vi "Result Datam.vi"() -> ()   [LabVIEW 2012]
uses:
  <vilib>/Analysis/NI_AALPro.lvlib
panel:
  out "Graph Polarizer":cluster{dbl[], dbl[]}[](graph)
  in  "Polarizer and Analyser Scan":refnum<user-event>
  in  "Polarizer Scan":refnum<user-event>
  in  "Make this a motor null":refnum<user-event>
  in  "Panel Clouse and Stop":refnum<user-event>
  in  "Minimum Absolute Null":i32(listbox)
  in  "Table Absolute Null":i32(listbox)
  in  "Table Polarizer":i32(listbox)
  in  "Event Polarizer":refnum<user-event>
  in  "stop":bool
  out "XY Absolute Null":cluster{dbl[], dbl[]}[](graph)
  # "Polarizer"
  # "Absolute null"
  # "Minimum"
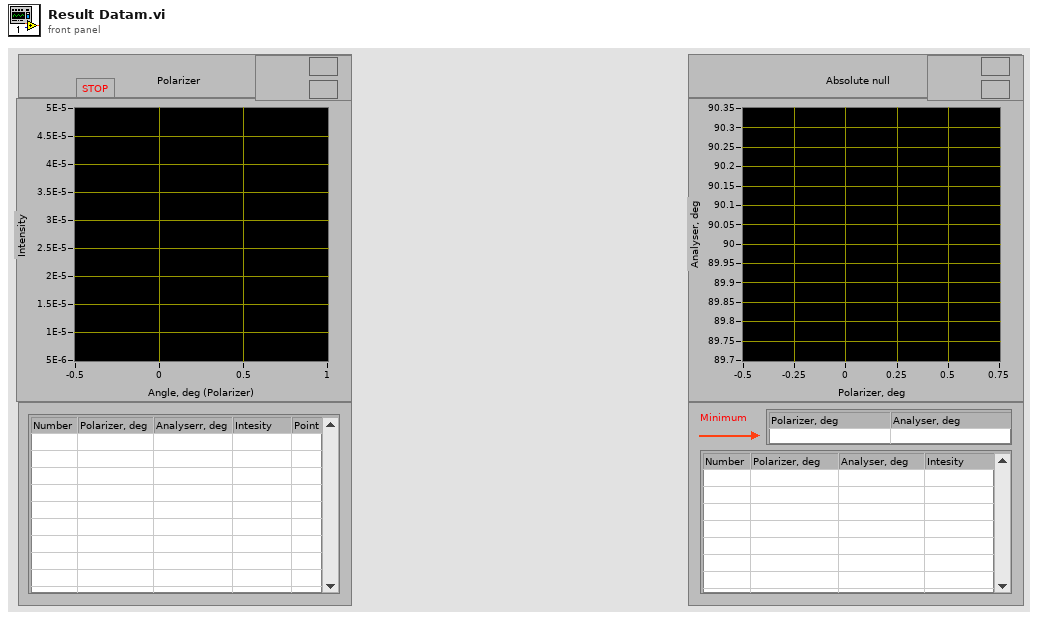
[diagram p1: front panel]
types:
  T1 = cluster{"Counter Pol":i32, "Counter A":i32, "Number Graph Pol":i32, "Number Graph A":i32, "Counter Abs Null":i32, "Pol Abs null deg":dbl, "A Abs null deg":dbl}
  T2 = cluster{"Kol-vo":i32, "Analyser":dbl, dbl[], dbl[], dbl[]}
  T3 = cluster{"Kol-vo":i32, "Analyser":dbl, dbl[], dbl[], dbl[]}[]
  T4 = cluster{"Kol-vo":i32, "Polarizer":dbl, dbl[], dbl[], dbl[]}
  T5 = cluster{"Kol-vo":i32, "Polarizer":dbl, dbl[], dbl[], dbl[]}[]
  T6 = enum32{"SVD", "Givens", "Givens2", "Householder", "LU Decomposition", "Cholesky"}
  T7 = cluster{"Pol Abs null deg":dbl, "A Abs null deg":dbl}
  T8 = cluster{"Kol-vo":i32, "Analyser":dbl, dbl[], dbl[], "Best Polynomial Fit":dbl[]}
  T9 = cluster{"Kol-vo":i32, "Polarizer":dbl, dbl[], dbl[], "Best Polynomial Fit":dbl[]}
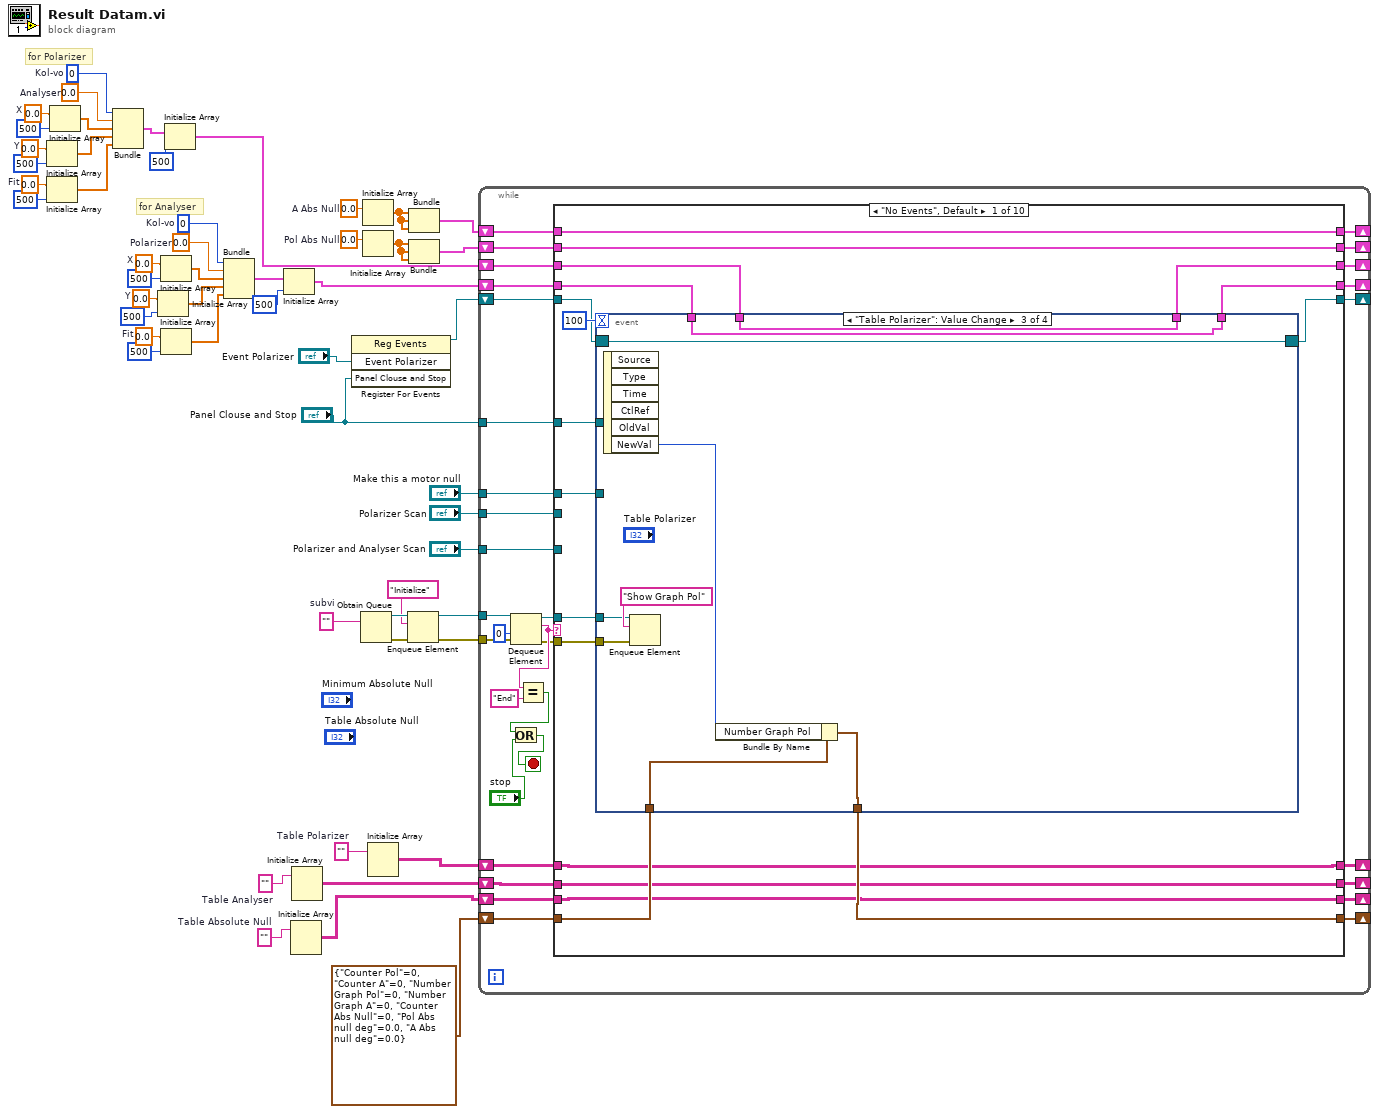
[diagram p0: block diagram]
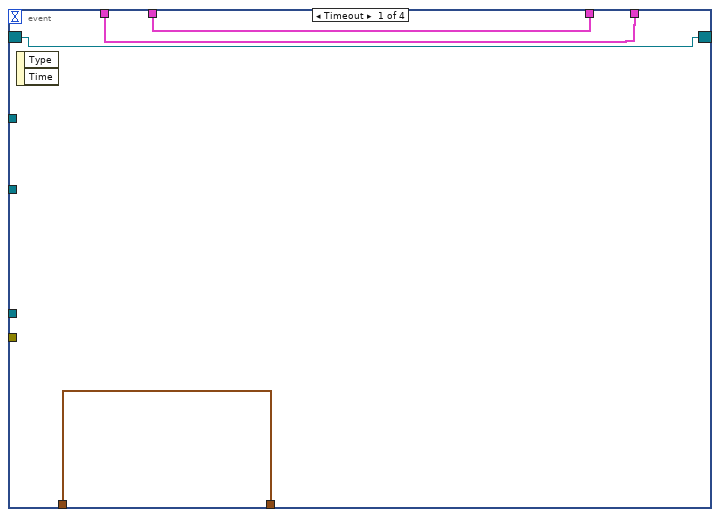
[diagram p2: hidden frame]
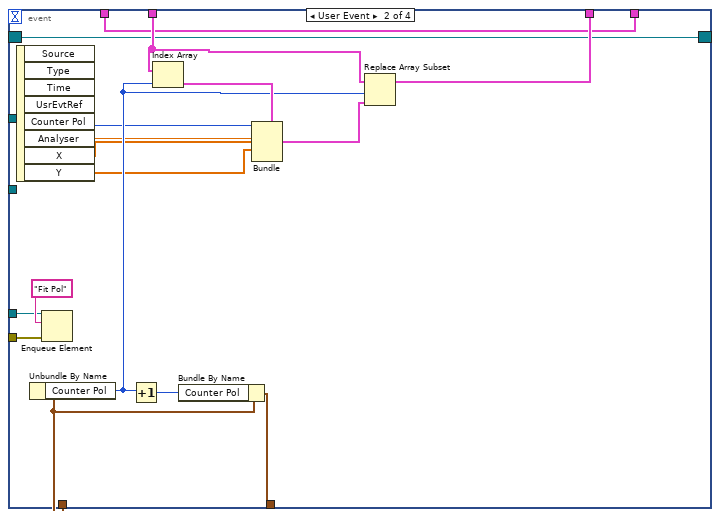
[diagram p3: hidden frame]
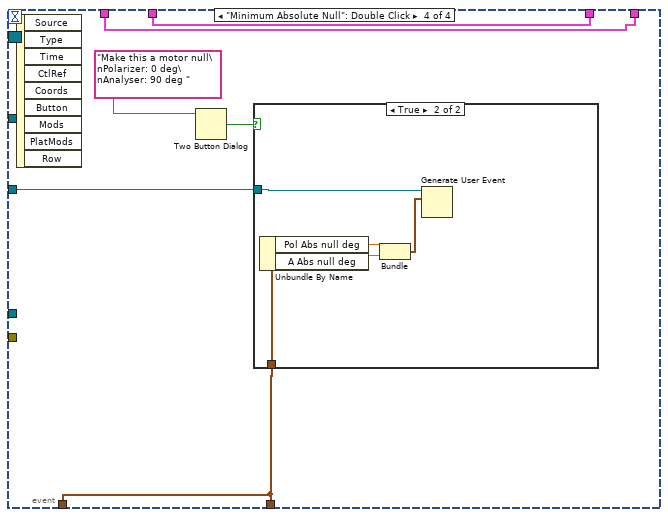
[diagram p4: hidden frame]
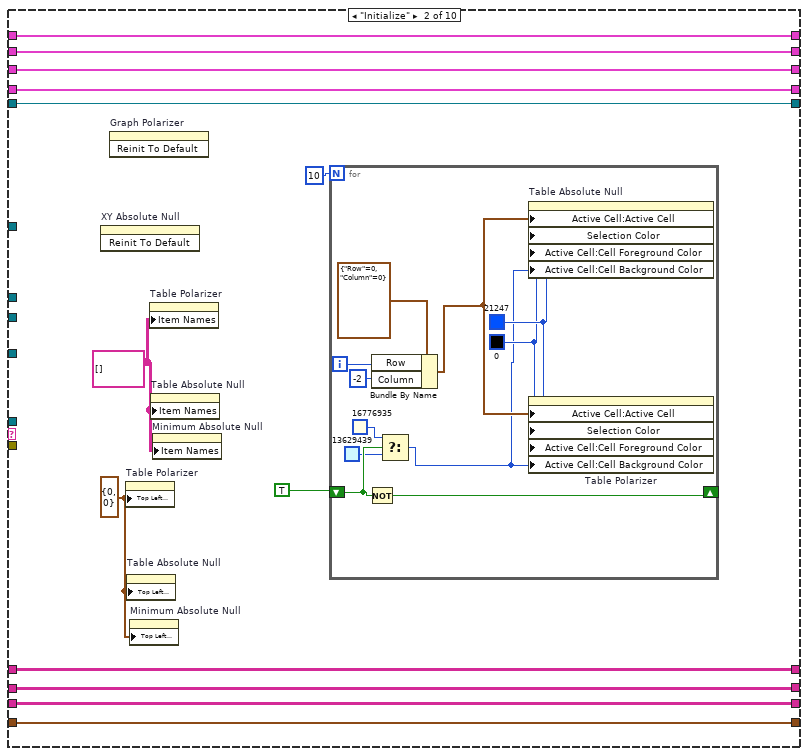
[diagram p6: hidden frame]
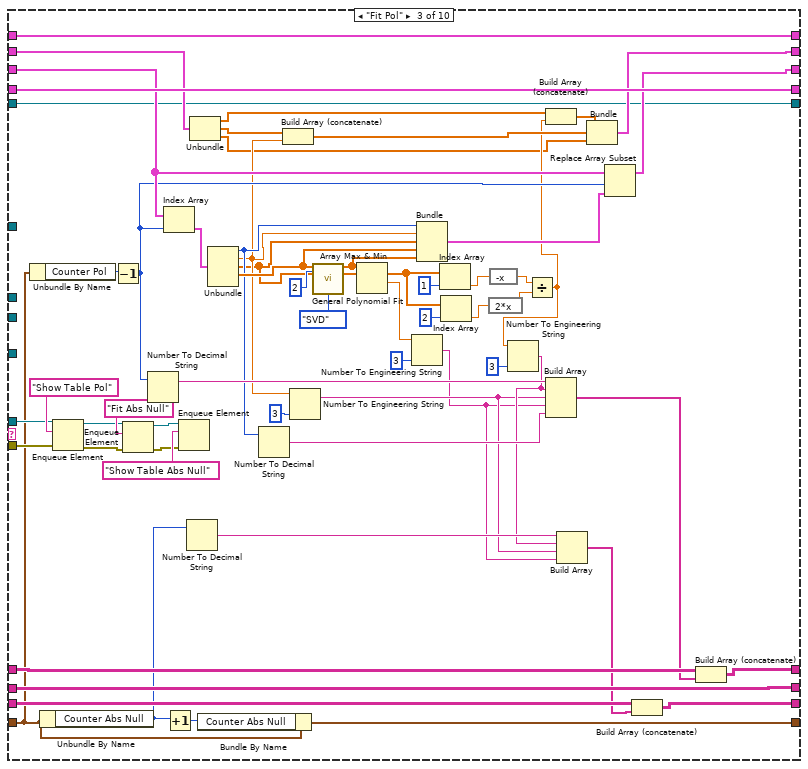
[diagram p7: hidden frame]
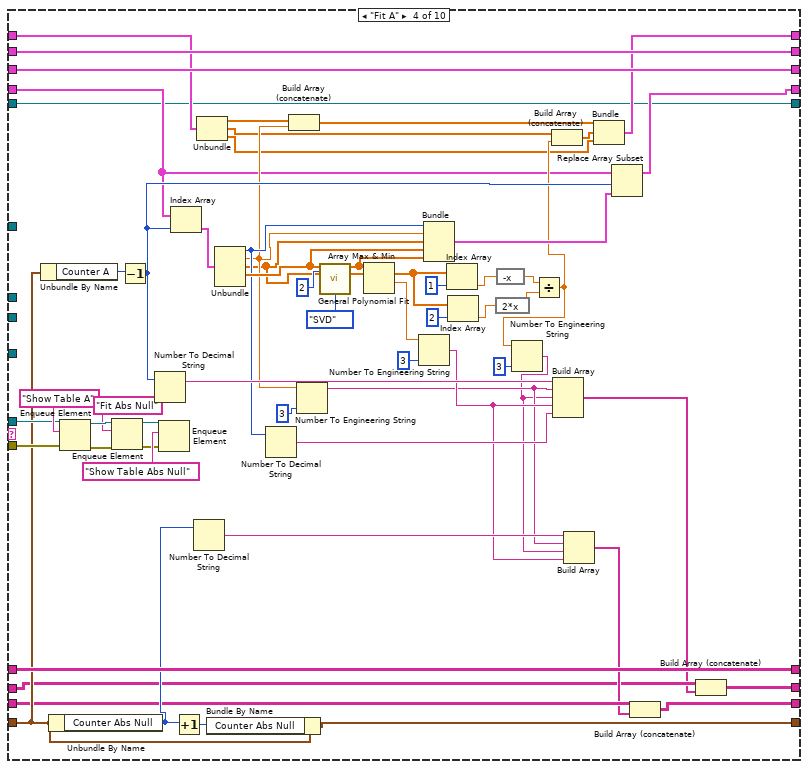
[diagram p8: hidden frame]
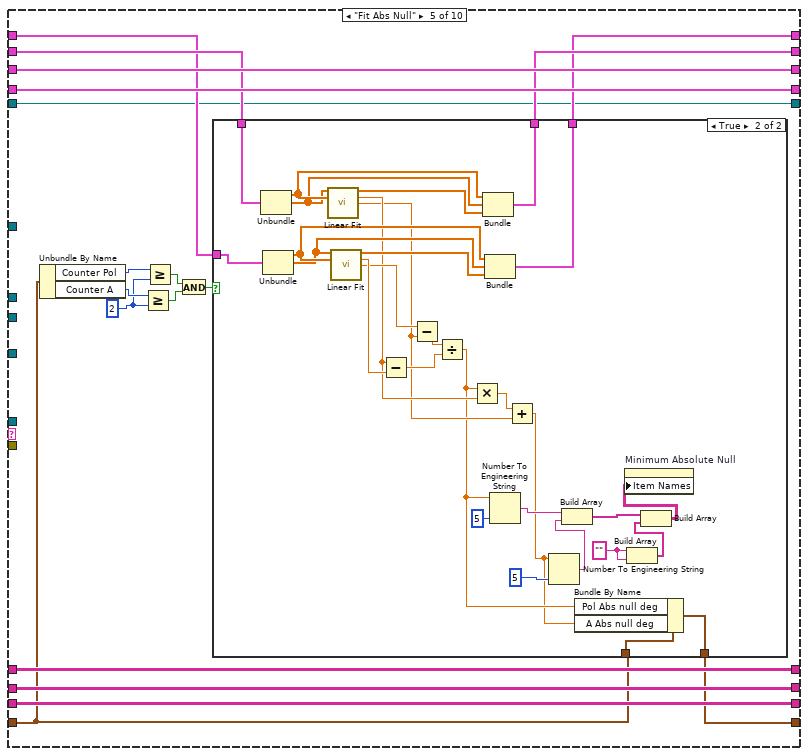
[diagram p9: hidden frame]
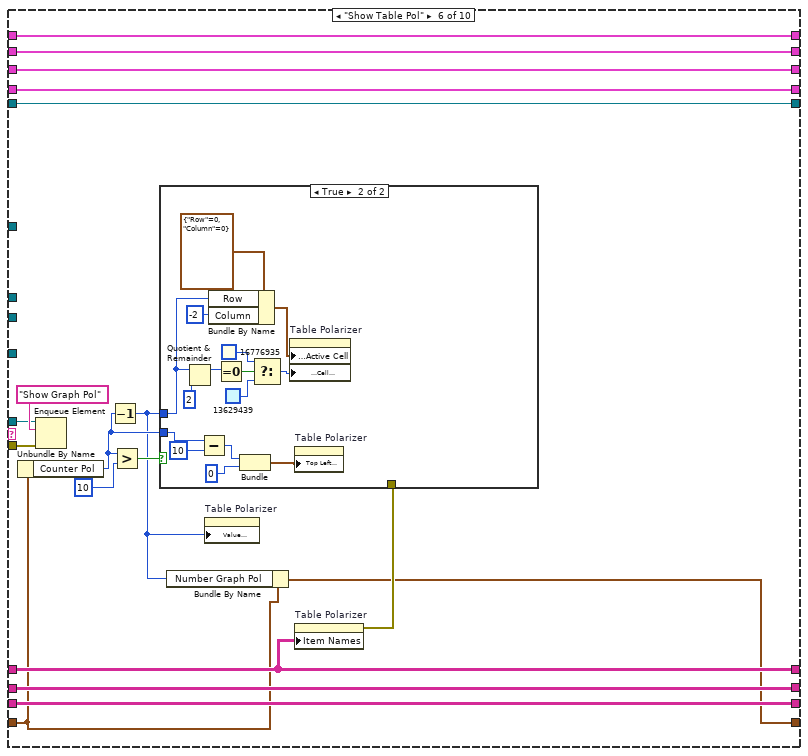
[diagram p11: hidden frame]
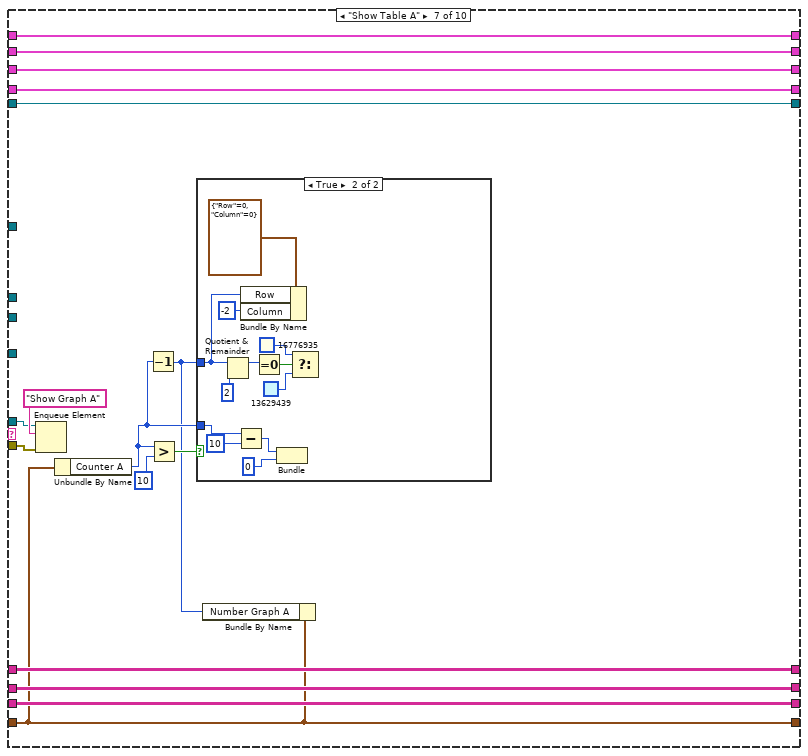
[diagram p13: hidden frame]
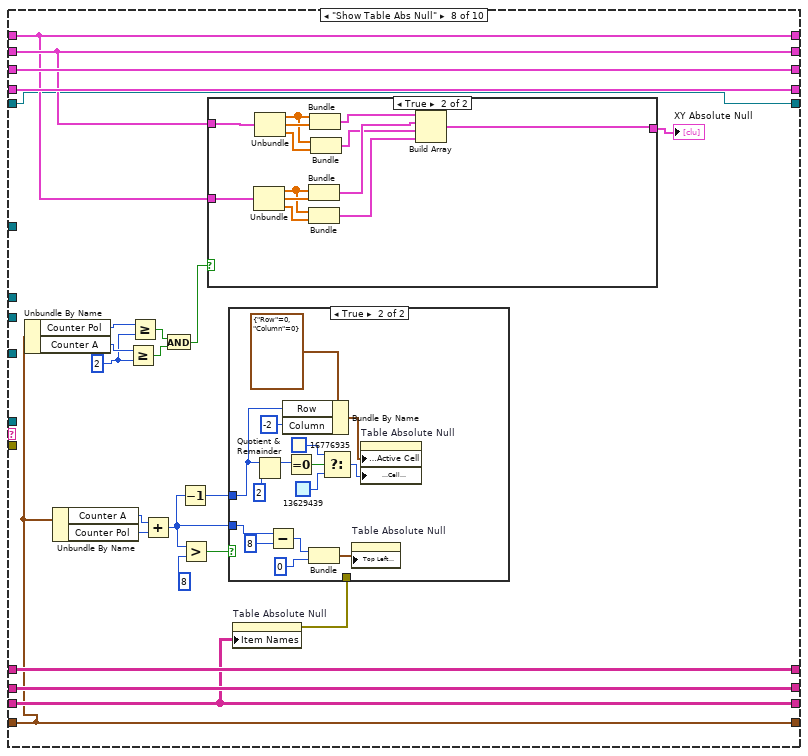
[diagram p15: hidden frame]
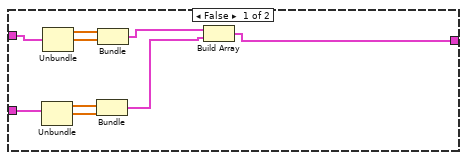
[diagram p17: hidden frame]
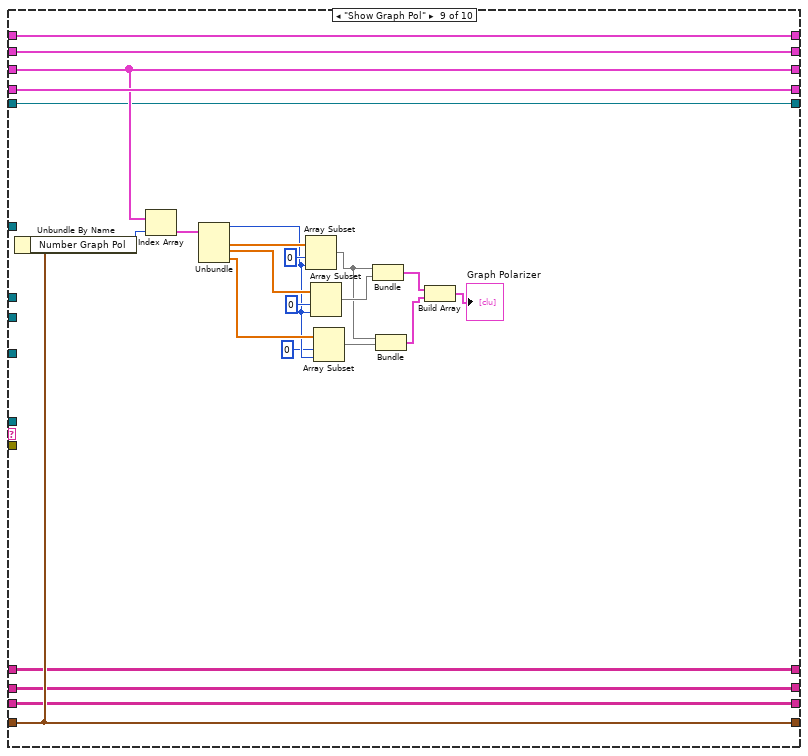
[diagram p18: hidden frame]
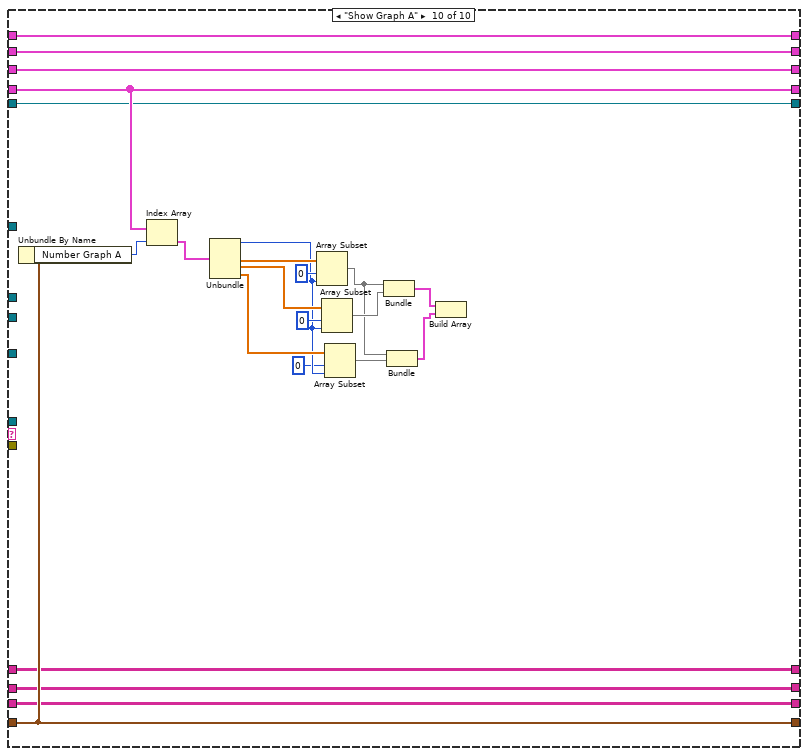
[diagram p19: hidden frame]
diagram:
  w9 = 0.0  # A Abs Null
  w11 = 0.0  # Pol Abs Null
  w13 = ""  # Table Absolute Null
  w15 = ""  # Table Analyser
  w17 = ""  # Table Polarizer
  w20 = 0.0  # Fit
  w23 = 0.0  # Fit
  w35 = 0  # Kol-vo
  w37 = 0.0  # Y
  w34 = 0.0  # Polarizer
  w39 = 0.0  # X
  w43 = 0  # Kol-vo
  w45 = 0.0  # Y
  w42 = 0.0  # Analyser
  w47 = 0.0  # X
  w53 = ""  # subvi
  # "for Analyser"
  # "for Polarizer"
  n1 = Initialize Array(w45, 500 ("dimension size")) -> (w40:dbl[])
  n2 = Initialize Array(w23, 500 ("dimension size")) -> (w21:dbl[])
  n3 = Initialize Array(w47, 500 ("dimension size")) -> (w41:dbl[])
  n4 = Bundle("Kol-vo"=w43, "Analyser"=w42, w41, w40, w21) -> (w29:T2)  [unwired: 1 in]
  n5 = Initialize Array(w37, 500 ("dimension size")) -> (w32:dbl[])
  n6 = Initialize Array(w39, 500 ("dimension size")) -> (w33:dbl[])
  n7 = Initialize Array(w20, 500 ("dimension size")) -> (w18:dbl[])
  n8 = Initialize Array(w29, 500 ("dimension size")) -> (w27:T3)
  n9 = Bundle("Kol-vo"=w35, "Polarizer"=w34, w33, w32, w18) -> (w31:T4)  [unwired: 1 in]
  n10 = Initialize Array(w31, 500 ("dimension size")) -> (w26:T5)
  n11 = Initialize Array(w13) -> (w12:string[][])  [unwired: 2 in]
  n12 = Initialize Array(w15) -> (w14:string[][])  [unwired: 2 in]
  n13 = register-events("Event Polarizer", "Panel Clouse and Stop") -> (reference out=w5:refnum<event-registration>)  [unwired: 2 in, 1 out]
  n14 = Obtain Queue(element data type=w53) -> (queue out=w52:refnum<queue>, error out=w50:errorcluster)  [unwired: 4 in, 1 out]
  n15 = Initialize Array(w9) -> (w7:dbl[])  [unwired: 1 in]
  n16 = Initialize Array(w11) -> (w6:dbl[])  [unwired: 1 in]
  n17 = Initialize Array(w17) -> (w16:string[][])  [unwired: 2 in]
  n18 = Enqueue Element(queue=w52, element="Initialize", error in (no error)=w50) -> (queue out=w49:refnum<queue>, error out=w48:errorcluster)  [unwired: 1 in, 1 out]
  n19 = Bundle(w7, w7, w7) -> (w8:cluster{dbl[], dbl[], dbl[]})  [unwired: 1 in]
  n20 = Bundle(w6, w6, w6) -> (w10:cluster{dbl[], dbl[], dbl[]})  [unwired: 1 in]
  n21 = while {
    tunnel: w49 -> [w83]
    tunnel: w48 -> [w82]
    shift-right: [w71] -> _
    shift-left: w27 -> [w74]
    shift-right: [w70] -> _
    shift-left: w26 -> [w75]
    shift-right: [w72] -> _
    shift-left: T1 {"Counter Pol"=0, "Counter A"=0, "Number Graph Pol"=0, "Number Graph A"=0, "Counter Abs Null"=0, "Pol Abs null deg"=0.0, "A Abs null deg"=0.0} -> [w73]
    shift-right: [w68] -> _
    shift-left: w16 -> [w69]
    shift-right: [w66] -> _
    shift-left: w14 -> [w67]
    shift-right: [w64] -> _
    shift-left: w12 -> [w65]
    shift-right: [w62] -> _
    shift-left: w10 -> [w63]
    shift-right: [w60] -> _
    shift-left: w8 -> [w61]
    shift-right: [w57] -> _
    shift-left: w5 -> [w59]
    tunnel: "Panel Clouse and Stop" -> [w58]
    tunnel: "Make this a motor null" -> [w56]
    tunnel: "Polarizer Scan" -> [w55]
    tunnel: "Polarizer and Analyser Scan" -> [w54]
    stop <- w78 stop-if-true
    n22 = Dequeue Element(queue=w83, timeout in ms (-1)=0, error in (no error)=w82) -> (queue out=w76:refnum<queue>, element=w81:string, error out=w77:errorcluster)  [unwired: 1 out]
    n23 = Equal?(x=w81, y="End") -> (x = y?=w80:bool)
    n24 = Or(x=w80, y="stop") -> (x .or. y?=w78:bool)
    n25 = case shown="\"No Events\", Default" w81 {
      tunnel: w77 -> [w102 _ w226 w257 _ w343 w378 _ _ _]
      tunnel: w76 -> [w101 _ w227 w258 _ w342 w377 _ _ _]
      tunnel: w75 -> [w96 w157 w229 w252 w299 w357 w386 w422 w485 w506]
      tunnel: w74 -> [w100 w156 w224 w289 w298 w358 w387 w421 w484 w507]
      tunnel: w73 -> [w99 w154 w202 w255 w292 w347 w376 w409 w483 w505]
      tunnel: [w98 w154 w204 w253 w291 w346 w376 w409 w483 w505] -> w72
      tunnel: [w97 w156 w218 w289 w298 w358 w387 w421 w484 w507] -> w71
      tunnel: [w95 w157 w229 w249 w299 w357 w386 w422 w485 w506] -> w70
      tunnel: w69 -> [w94 w155 w217 w288 w306 w356 w385 w423 w475 w504]
      tunnel: [w94 w155 w216 w288 w306 w356 w385 w423 w475 w504] -> w68
      tunnel: [w93 w153 w208 w244 w307 w355 w383 w424 w474 w503] -> w66
      tunnel: w67 -> [w93 w153 w208 w245 w307 w355 w383 w424 w474 w503]
      tunnel: [w92 w152 w205 w246 w308 w354 w384 w420 w473 w502] -> w64
      tunnel: w65 -> [w92 w152 w206 w248 w308 w354 w384 w420 w473 w502]
      tunnel: [w91 w151 w185 w290 w296 w353 w388 w419 w472 w501] -> w62
      tunnel: w63 -> [w91 w151 w191 w290 w297 w353 w388 w419 w472 w501]
      tunnel: [w90 w150 w207 w250 w294 w352 w389 w418 w471 w500] -> w60
      tunnel: w61 -> [w90 w150 w207 w251 w295 w352 w389 w418 w471 w500]
      tunnel: w59 -> [w89 w145 w169 w230 w293 w341 w374 w403 w462 w486]
      tunnel: w58 -> [w88 _ _ _ _ _ _ _ _ _]
      tunnel: [w87 w145 w169 w230 w293 w341 w374 w403 w462 w486] -> w57
      tunnel: w56 -> [w86 _ _ _ _ _ _ _ _ _]
      tunnel: w55 -> [_ _ _ _ _ _ _ _ _ _]
      tunnel: w54 -> [_ _ _ _ _ _ _ _ _ _]
      frame "No Events", Default {
        n26 = event shown="[2] \"Table Polarizer\": Value Change" {
          selector: w89 -> [w104 w108 w125 _]
          dyn-events: [w104 w108 w125 _] -> w87
          timeout: 100 -> [_ _ _ _]
          tunnel: w102 -> [_ w110 w130 _]
          tunnel: w101 -> [_ w109 w129 _]
          tunnel: w100 -> [w107 w120 w133 w139]
          tunnel: w99 -> [w105 w123 w127 w134]
          tunnel: [w105 w124 w128 w134] -> w98
          tunnel: [w107 w117 w133 w139] -> w97
          tunnel: w96 -> [w106 w116 w132 w138]
          tunnel: [w106 w116 w132 w138] -> w95
          tunnel: w88 -> [_ _ _ _]
          tunnel: w86 -> [_ _ _ w135]
          event Timeout {
            n27 = event-data() -> ()  [unwired: 1 in, 2 out]
          }
          event User Event {
            n28 = event-data() -> ("Counter Pol"=w112:i32, "Analyser"=w113:dbl, "X"=w114:dbl[], "Y"=w115:dbl[])  [unwired: 1 in, 4 out]
            n29 = Unbundle By Name(w123) -> ("Counter Pol"=w119:i32)
            n30 = Enqueue Element(queue=w109, element="Fit Pol", error in (no error)=w110) -> ()  [unwired: 1 in, 3 out]
            n31 = Increment(x=w119) -> (x+1=w122:i32)
            n32 = Index Array(array=w120, index=w119) -> (element=w121:T2)
            n33 = Bundle By Name(cluster=w123, "Counter Pol"=w122) -> (w124:T1)
            n34 = Bundle(cluster=w121, "Kol-vo"=w112, "Analyser"=w113, w114, w115) -> (w118:T2)  [unwired: 1 in]
            n35 = Replace Array Subset(array=w120, new element=w118, index=w119) -> (w117:T3)
          }
          event "Table Polarizer": Value Change {
            n36 = event-data() -> ("NewVal"=w126:i32)  [unwired: 1 in, 5 out]
            n37 = Enqueue Element(queue=w129, element="Show Graph Pol", error in (no error)=w130) -> ()  [unwired: 1 in, 3 out]
            n38 = Bundle By Name(cluster=w127, "Number Graph Pol"=w126) -> (w128:T1)
          }
          event "Minimum Absolute Null": Double Click {
            n39 = event-data() -> ()  [unwired: 1 in, 9 out]
            n40 = Two Button Dialog(message="Make this a motor null\nPolarizer: 0 deg\nAnalyser: 90 deg ") -> (T button?=w136:bool)  [unwired: 2 in]
            n41 = case shown="True" w136 {
              tunnel: w135 -> [_ w143]
              tunnel: w134 -> [_ w144]
              frame False {
              }
              frame True {
                n42 = Unbundle By Name(w144) -> ("Pol Abs null deg"=w142:dbl, "A Abs null deg"=w141:dbl)
                n43 = Bundle("Pol Abs null deg"=w142, "A Abs null deg"=w141) -> (w140:T7)  [unwired: 1 in]
                n44 = Generate User Event(user event=w143, event data cluster=w140) -> ()  [unwired: 1 in, 2 out]
              }
            }
          }
        }
      }
      frame "Initialize" {
        w147 = cluster{"Row":u32, "Column":u32} {"Row"=0, "Column"=0} ("Top Left Visible Cell")
        w146 = string[][] [] ("Item Names")
        n45 = invoke on="XY Absolute Null" class="XYGraph (strict)" method="Reinit To Default"() -> ()  [unwired: 3 in, 3 out]
        n46 = invoke on="Graph Polarizer" class="XYGraph (strict)" method="Reinit To Default"() -> ()  [unwired: 3 in, 3 out]
        n47 = property on="Table Polarizer" class="MCListbox (strict)"("Top Left Visible Cell"=w147) -> ()  [unwired: 2 in, 2 out]
        n48 = property on="Table Absolute Null" class="MCListbox (strict)"("Top Left Visible Cell"=w147) -> ()  [unwired: 2 in, 2 out]
        n49 = property on="Minimum Absolute Null" class="MCListbox (strict)"("Top Left Visible Cell"=w147) -> ()  [unwired: 2 in, 2 out]
        n50 = property on="Table Polarizer" class="MCListbox (strict)"("Item Names"=w146) -> ()  [unwired: 2 in, 2 out]
        n51 = property on="Table Absolute Null" class="MCListbox (strict)"("Item Names"=w146) -> ()  [unwired: 2 in, 2 out]
        n52 = property on="Minimum Absolute Null" class="MCListbox (strict)"("Item Names"=w146) -> ()  [unwired: 2 in, 2 out]
        n53 = for {
          N: 10 -> [_]
          shift-right: [w165] -> _
          shift-left: TRUE -> [w164]
          i -> [w167]
          w159 = u32 0 ("Color Box")
          w160 = u32 21247 ("Color Box")
          n54 = Not(x=w164) -> (.not. x?=w165:bool)
          n55 = Bundle By Name(cluster=cluster{"Row":i32, "Column":i32} {"Row"=0, "Column"=0}, "Row"=w167, "Column"=-2) -> (w161:cluster{"Row":i32, "Column":i32})
          n56 = Select(t=u32 16776935 ("Color Box"), s=w164, f=u32 13629439 ("Color Box")) -> (s? t:f=w158:u32)
          n57 = property on="Table Absolute Null" class="MulticolumnListbox (strict)"("Active Cell:Active Cell"=w161, "Selection Color"=w160, "Active Cell:Cell Foreground Color"=w159, "Active Cell:Cell Background Color"=w158) -> ()  [unwired: 2 in, 2 out]
          n58 = property on="Table Polarizer" class="MulticolumnListbox (strict)"("Active Cell:Active Cell"=w161, "Selection Color"=w160, "Active Cell:Cell Foreground Color"=w159, "Active Cell:Cell Background Color"=w158) -> ()  [unwired: 2 in, 2 out]
        }
      }
      frame "Fit Pol" {
        n59 = Unbundle By Name(w202) -> ("Counter Pol"=w225:i32)
        n60 = Unbundle By Name(w202) -> ("Counter Abs Null"=w201:i32)
        n61 = Enqueue Element(queue=w227, element="Show Table Pol", error in (no error)=w226) -> (queue out=w173:refnum<queue>, error out=w172:errorcluster)  [unwired: 1 in, 1 out]
        n62 = Decrement(x=w225) -> (x-1=w215:i32)
        n63 = Enqueue Element(queue=w173, element="Fit Abs Null", error in (no error)=w172) -> (queue out=w170:refnum<queue>, error out=w171:errorcluster)  [unwired: 1 in, 1 out]
        n64 = Number To Decimal String(number=w215) -> (decimal integer string=w214:string)  [unwired: 1 in]
        n65 = Index Array(array=w224, index=w215) -> (element=w221:T2)
        n66 = Increment(x=w201) -> (x+1=w203:i32)
        n67 = Enqueue Element(queue=w170, element="Show Table Abs Null", error in (no error)=w171) -> ()  [unwired: 1 in, 3 out]
        n68 = Number To Decimal String(number=w201) -> (decimal integer string=w200:string)  [unwired: 1 in]
        n69 = Unbundle(w191) -> (w190:dbl[], w189:dbl[], w175:dbl[])
        n70 = Bundle By Name(cluster=w202, "Counter Abs Null"=w203) -> (w204:T1)
        n71 = Unbundle(w221) -> ("Kol-vo"=w211:i32, "Analyser"=w188:dbl, w184:dbl[], w220:dbl[])  [unwired: 1 out]
        n72 = Number To Decimal String(number=w211) -> (decimal integer string=w210:string)  [unwired: 1 in]
        n73 = Build Array (concatenate)(w189, w188) -> (w186:dbl[])
        n74 = Number To Engineering String(2:i16 3 ("precision (6)"), 4:w188) -> (0:w198:string)  [unwired: 2 in]
        n75 = call <vilib>:"General Polynomial Fit.vi"("Y"=w220, "polynomial order"=2, "X"=w184, "algorithm"=T6."SVD") -> ("Best Polynomial Fit"=w213:dbl[], "Polynomial Coefficients"=w177:dbl[])  [unwired: 8 in, 2 out]
        n76 = Array Max & Min(array=w213) -> (min value=w212:dbl)  [unwired: 3 out]
        n77 = Number To Engineering String(2:i16 3 ("precision (6)"), 4:w212) -> (0:w197:string)  [unwired: 2 in]
        n78 = Bundle("Kol-vo"=w211, "Analyser"=w188, w184, w220, "Best Polynomial Fit"=w213) -> (w219:T8)  [unwired: 1 in]
        n79 = Index Array(array=w177, index=1) -> (element=w180:dbl)
        n80 = Index Array(array=w177, index=2) -> (element=w181:dbl)
        n81 = expression code="2*x"(w181) -> (w182:dbl)
        n82 = expression code="-x"(w180) -> (w183:dbl)
        n83 = Divide(x=w183, y=w182) -> (x/y=w176:dbl)
        n84 = Number To Engineering String(2:i16 3 ("precision (6)"), 4:w176) -> (0:w199:string)  [unwired: 2 in]
        n85 = Build Array (concatenate)(w190, w176) -> (w187:dbl[])
        n86 = Build Array(w214, w199, w198, w197, w210) -> (w209:string[])
        n87 = Build Array(w200, w199, w198, w197) -> (w196:string[])
        n88 = Bundle(w187, w186, w175) -> (w185:cluster{dbl[], dbl[], dbl[]})  [unwired: 1 in]
        n89 = Replace Array Subset(array=w224, new element=w219, index=w215) -> (w218:T3)
        n90 = Build Array (concatenate)(w206, w196) -> (w205:string[][])
        n91 = Build Array (concatenate)(w217, w209) -> (w216:string[][])
      }
      frame "Fit A" {
        n92 = Unbundle By Name(w255) -> ("Counter A"=w286:i32)
        n93 = Unbundle By Name(w255) -> ("Counter Abs Null"=w254:i32)
        n94 = Enqueue Element(queue=w258, element="Show Table A", error in (no error)=w257) -> (queue out=w236:refnum<queue>, error out=w235:errorcluster)  [unwired: 1 in, 1 out]
        n95 = Enqueue Element(queue=w236, element="Fit Abs Null", error in (no error)=w235) -> (queue out=w232:refnum<queue>, error out=w233:errorcluster)  [unwired: 1 in, 1 out]
        n96 = Decrement(x=w286) -> (x-1=w280:i32)
        n97 = Number To Decimal String(number=w280) -> (decimal integer string=w279:string)  [unwired: 1 in]
        n98 = Enqueue Element(queue=w232, element="Show Table Abs Null", error in (no error)=w233) -> ()  [unwired: 1 in, 3 out]
        n99 = Index Array(array=w252, index=w280) -> (element=w283:T4)
        n100 = Increment(x=w254) -> (x+1=w256:i32)
        n101 = Number To Decimal String(number=w254) -> (decimal integer string=w274:string)  [unwired: 1 in]
        n102 = Unbundle(w251) -> (w242:dbl[], w240:dbl[], w231:dbl[])
        n103 = Bundle By Name(cluster=w255, "Counter Abs Null"=w256) -> (w253:T1)
        n104 = Unbundle(w283) -> ("Kol-vo"=w276:i32, "Polarizer"=w268:dbl, w267:dbl[], w282:dbl[])  [unwired: 1 out]
        n105 = Number To Decimal String(number=w276) -> (decimal integer string=w275:string)  [unwired: 1 in]
        n106 = Build Array (concatenate)(w242, w268) -> (w241:dbl[])
        n107 = Number To Engineering String(2:i16 3 ("precision (6)"), 4:w268) -> (0:w238:string)  [unwired: 2 in]
        n108 = call <vilib>:"General Polynomial Fit.vi"("Y"=w282, "polynomial order"=2, "X"=w267, "algorithm"=T6."SVD") -> ("Best Polynomial Fit"=w278:dbl[], "Polynomial Coefficients"=w260:dbl[])  [unwired: 8 in, 2 out]
        n109 = Array Max & Min(array=w278) -> (min value=w277:dbl)  [unwired: 3 out]
        n110 = Number To Engineering String(2:i16 3 ("precision (6)"), 4:w277) -> (0:w273:string)  [unwired: 2 in]
        n111 = Bundle("Kol-vo"=w276, "Polarizer"=w268, w267, w282, "Best Polynomial Fit"=w278) -> (w281:T9)  [unwired: 1 in]
        n112 = Index Array(array=w260, index=1) -> (element=w263:dbl)
        n113 = Index Array(array=w260, index=2) -> (element=w264:dbl)
        n114 = expression code="2*x"(w264) -> (w265:dbl)
        n115 = expression code="-x"(w263) -> (w266:dbl)
        n116 = Divide(x=w266, y=w265) -> (x/y=w259:dbl)
        n117 = Number To Engineering String(2:i16 3 ("precision (6)"), 4:w259) -> (0:w237:string)  [unwired: 2 in]
        n118 = Build Array (concatenate)(w240, w259) -> (w239:dbl[])
        n119 = Build Array(w279, w238, w237, w273, w275) -> (w243:string[])
        n120 = Build Array(w274, w238, w237, w273) -> (w247:string[])
        n121 = Bundle(w241, w239, w231) -> (w250:cluster{dbl[], dbl[], dbl[]})  [unwired: 1 in]
        n122 = Replace Array Subset(array=w252, new element=w281, index=w280) -> (w249:T5)
        n123 = Build Array (concatenate)(w248, w247) -> (w246:string[][])
        n124 = Build Array (concatenate)(w245, w243) -> (w244:string[][])
      }
      frame "Fit Abs Null" {
        w303 = 2 ("y")
        n125 = Unbundle By Name(w292) -> ("Counter Pol"=w304:i32, "Counter A"=w305:i32)
        n126 = Greater Or Equal?(x=w305, y=w303) -> (x >= y?=w301:bool)
        n127 = Greater Or Equal?(x=w304, y=w303) -> (x >= y?=w302:bool)
        n128 = And(x=w302, y=w301) -> (x .and. y?=w300:bool)
        n129 = case shown="True" w300 {
          tunnel: w297 -> [w311 w340]
          tunnel: [w311 w336] -> w296
          tunnel: w295 -> [w310 w335]
          tunnel: [w310 w331] -> w294
          tunnel: w292 -> [w309 w315]
          tunnel: [w309 w312] -> w291
          frame False {
          }
          frame True {
            w316 = ""
            n130 = Unbundle(w340) -> (w338:dbl[], w337:dbl[])  [unwired: 1 out]
            n131 = Unbundle(w335) -> (w333:dbl[], w332:dbl[])  [unwired: 1 out]
            n132 = call <vilib>:"Linear Fit.vi"("Y"=w337, "X"=w338) -> ("Best Linear Fit"=w339:dbl[], "slope"=w326:dbl, "intercept"=w324:dbl)  [unwired: 9 in, 2 out]
            n133 = call <vilib>:"Linear Fit.vi"("Y"=w332, "X"=w333) -> ("Best Linear Fit"=w334:dbl[], "slope"=w330:dbl, "intercept"=w329:dbl)  [unwired: 9 in, 2 out]
            n134 = Subtract(x=w326, y=w330) -> (x-y=w327:dbl)
            n135 = Subtract(x=w329, y=w324) -> (x-y=w328:dbl)
            n136 = Divide(x=w328, y=w327) -> (x/y=w314:dbl)
            n137 = Multiply(x=w314, y=w326) -> (x*y=w325:dbl)
            n138 = Bundle(w338, w337, "Best Linear Fit"=w339) -> (w336:cluster{dbl[], dbl[], "Best Linear Fit":dbl[]})  [unwired: 1 in]
            n139 = Bundle(w333, w332, "Best Linear Fit"=w334) -> (w331:cluster{dbl[], dbl[], "Best Linear Fit":dbl[]})  [unwired: 1 in]
            n140 = Number To Engineering String(2:i16 5 ("precision (6)"), 4:w314) -> (0:w321:string)  [unwired: 2 in]
            n141 = Add(x=w325, y=w324) -> (x+y=w313:dbl)
            n142 = Number To Engineering String(2:i16 5 ("precision (6)"), 4:w313) -> (0:w320:string)  [unwired: 2 in]
            n143 = Build Array(w321, w320) -> (w319:string[])
            n144 = Bundle By Name(cluster=w315, "Pol Abs null deg"=w314, "A Abs null deg"=w313) -> (w312:T1)
            n145 = Build Array(w316, w316) -> (w318:string[])
            n146 = Build Array(w319, w318) -> (w317:string[][])
            n147 = property on="Minimum Absolute Null" class="MCListbox (strict)"("Item Names"=w317) -> ()  [unwired: 2 in, 2 out]
          }
        }
      }
      frame "Show Table Pol" {
        n148 = Unbundle By Name(w347) -> ("Counter Pol"=w348:i32)
        n149 = Enqueue Element(queue=w342, element="Show Graph Pol", error in (no error)=w343) -> ()  [unwired: 1 in, 3 out]
        n150 = Decrement(x=w348) -> (x-1=w345:i32)
        n151 = Greater?(x=w348, y=10) -> (0:w350:bool)
        n152 = Bundle By Name(cluster=w347, "Number Graph Pol"=w345) -> (w346:T1)
        n153 = property on="Table Polarizer" class="MCListbox (strict)"("Value (Signaling)"=w345) -> ()  [unwired: 2 in, 2 out]
        n154 = property on="Table Polarizer" class="MCListbox (strict)"("Item Names"=w356) -> (error out=w349:errorcluster)  [unwired: 2 in, 1 out]
        n155 = case shown="True" w350 {
          tunnel: w348 -> [_ w373]
          tunnel: w349 -> [_ _]
          tunnel: w345 -> [_ w360]
          frame False {
          }
          frame True {
            n156 = Quotient & Remainder(x=w360, y=2) -> (x-y*floor(x/y)=w367:i32)  [unwired: 1 out]
            n157 = Subtract(x=w373, y=10) -> (x-y=w371:i32)
            n158 = Bundle By Name(cluster=cluster{"Row":i32, "Column":i32} {"Row"=0, "Column"=0}, "Row"=w360, "Column"=-2) -> (w359:cluster{"Row":i32, "Column":i32})
            n159 = Equal To 0?(x=w367) -> (x = 0?=w366:bool)
            n160 = Bundle(w371, 0) -> (w369:cluster{i32, i32})  [unwired: 1 in]
            n161 = Select(t=u32 16776935 ("Color Box"), s=w366, f=u32 13629439 ("Color Box")) -> (s? t:f=w363:u32)
            n162 = property on="Table Polarizer" class="MCListbox (strict)"("Active Cell:Active Cell"=w359, "Active Cell:Cell Background Color"=w363) -> ()  [unwired: 2 in, 2 out]
            n163 = property on="Table Polarizer" class="MCListbox (strict)"("Top Left Visible Cell"=w369) -> ()  [unwired: 2 in, 2 out]
          }
        }
      }
      frame "Show Table A" {
        n164 = Enqueue Element(queue=w377, element="Show Graph A", error in (no error)=w378) -> ()  [unwired: 1 in, 3 out]
        n165 = Unbundle By Name(w376) -> ("Counter A"=w380:i32)
        n166 = Decrement(x=w380) -> (x-1=w375:i32)
        n167 = Greater?(x=w380, y=10) -> (0:w381:bool)
        n168 = case shown="True" w381 {
          tunnel: w380 -> [_ w401]
          tunnel: w375 -> [_ w391]
          frame False {
          }
          frame True {
            n169 = Quotient & Remainder(x=w391, y=2) -> (x-y*floor(x/y)=w394:i32)  [unwired: 1 out]
            n170 = Subtract(x=w401, y=10) -> (x-y=w399:i32)
            n171 = Bundle By Name(cluster=cluster{"Row":i32, "Column":i32} {"Row"=0, "Column"=0}, "Row"=w391, "Column"=-2) -> ()  [unwired: 1 out]
            n172 = Equal To 0?(x=w394) -> (x = 0?=w395:bool)
            n173 = Bundle(w399, 0) -> ()  [unwired: 1 in, 1 out]
            n174 = Select(t=u32 16776935 ("Color Box"), s=w395, f=u32 13629439 ("Color Box")) -> ()  [unwired: 1 out]
          }
        }
        n175 = Bundle By Name(cluster=w376, "Number Graph A"=w375) -> ()  [unwired: 1 out]
      }
      frame "Show Table Abs Null" {
        w415 = 2 ("y")
        n176 = Unbundle By Name(w409) -> ("Counter Pol"=w416:i32, "Counter A"=w417:i32)
        n177 = Unbundle By Name(w409) -> ("Counter A"=w407:i32, "Counter Pol"=w408:i32)
        n178 = Greater Or Equal?(x=w417, y=w415) -> (x >= y?=w413:bool)
        n179 = Greater Or Equal?(x=w416, y=w415) -> (x >= y?=w414:bool)
        n180 = Add(x=w407, y=w408) -> (x+y=w406:i32)
        n181 = And(x=w414, y=w413) -> (x .and. y?=w412:bool)
        n182 = Decrement(x=w406) -> (x-1=w405:i32)
        n183 = Greater?(x=w406, y=8) -> (0:w410:bool)
        n184 = case shown="True" w412 {
          tunnel: w419 -> [w443 w461]
          tunnel: w418 -> [w442 w456]
          tunnel: [w440 w451] -> w402
          frame False {
            n185 = Unbundle(w442) -> (w444:dbl[], w445:dbl[])  [unwired: 1 out]
            n186 = Unbundle(w443) -> (w446:dbl[], w448:dbl[])  [unwired: 1 out]
            n187 = Bundle(w444, w445) -> (w441:cluster{dbl[], dbl[]})  [unwired: 1 in]
            n188 = Bundle(w446, w448) -> (w447:cluster{dbl[], dbl[]})  [unwired: 1 in]
            n189 = Build Array(w447, w441) -> (w440:cluster{dbl[], dbl[]}[])
          }
          frame True {
            n190 = Unbundle(w456) -> (w454:dbl[], w455:dbl[], w453:dbl[])
            n191 = Unbundle(w461) -> (w458:dbl[], w460:dbl[], w457:dbl[])
            n192 = Bundle(w454, w455) -> (w450:cluster{dbl[], dbl[]})  [unwired: 1 in]
            n193 = Bundle(w454, w453) -> (w452:cluster{dbl[], dbl[]})  [unwired: 1 in]
            n194 = Bundle(w458, w460) -> (w459:cluster{dbl[], dbl[]})  [unwired: 1 in]
            n195 = Bundle(w458, w457) -> (w449:cluster{dbl[], dbl[]})  [unwired: 1 in]
            n196 = Build Array(w459, w450, w449, w452) -> (w451:cluster{dbl[], dbl[]}[])
          }
        }
        "XY Absolute Null" <- w402
        n197 = property on="Table Absolute Null" class="MCListbox (strict)"("Item Names"=w420) -> (error out=w404:errorcluster)  [unwired: 2 in, 1 out]
        n198 = case shown="True" w410 {
          tunnel: w406 -> [_ w439]
          tunnel: w405 -> [_ w426]
          tunnel: w404 -> [_ _]
          frame False {
          }
          frame True {
            n199 = Quotient & Remainder(x=w426, y=2) -> (x-y*floor(x/y)=w431:i32)  [unwired: 1 out]
            n200 = Subtract(x=w439, y=8) -> (x-y=w437:i32)
            n201 = Bundle By Name(cluster=cluster{"Row":i32, "Column":i32} {"Row"=0, "Column"=0}, "Row"=w426, "Column"=-2) -> (w425:cluster{"Row":i32, "Column":i32})
            n202 = Equal To 0?(x=w431) -> (x = 0?=w432:bool)
            n203 = Bundle(w437, 0) -> (w435:cluster{i32, i32})  [unwired: 1 in]
            n204 = Select(t=u32 16776935 ("Color Box"), s=w432, f=u32 13629439 ("Color Box")) -> (s? t:f=w429:u32)
            n205 = property on="Table Absolute Null" class="MCListbox (strict)"("Top Left Visible Cell"=w435) -> ()  [unwired: 2 in, 2 out]
            n206 = property on="Table Absolute Null" class="MCListbox (strict)"("Active Cell:Active Cell"=w425, "Active Cell:Cell Background Color"=w429) -> ()  [unwired: 2 in, 2 out]
          }
        }
      }
      frame "Show Graph Pol" {
        n207 = Unbundle By Name(w483) -> ("Number Graph Pol"=w482:i32)
        n208 = Index Array(array=w484, index=w482) -> (element=w481:T2)
        n209 = Unbundle(w481) -> ("Kol-vo"=w469:i32, w480:dbl[], w478:dbl[], w470:dbl[])  [unwired: 1 out]
        n210 = Array Subset(array=w480, index=0, length=w469) -> (w467:dbl[])
        n211 = Array Subset(array=w478, index=0, length=w469) -> (w476:dbl[])
        n212 = Array Subset(array=w470, index=0, length=w469) -> (w466:dbl[])
        n213 = Bundle(w467, w476) -> (w464:cluster{dbl[], dbl[]})  [unwired: 1 in]
        n214 = Bundle(w467, w466) -> (w465:cluster{dbl[], dbl[]})  [unwired: 1 in]
        n215 = Build Array(w464, w465) -> (→"Graph Polarizer":cluster{dbl[], dbl[]}[])
      }
      frame "Show Graph A" {
        n216 = Unbundle By Name(w505) -> ("Number Graph A"=w508:i32)
        n217 = Index Array(array=w506, index=w508) -> (element=w487:T4)
        n218 = Unbundle(w487) -> ("Kol-vo"=w493:i32, w499:dbl[], w497:dbl[], w494:dbl[])  [unwired: 1 out]
        n219 = Array Subset(array=w499, index=0, length=w493) -> (w491:dbl[])
        n220 = Array Subset(array=w497, index=0, length=w493) -> (w495:dbl[])
        n221 = Array Subset(array=w494, index=0, length=w493) -> (w490:dbl[])
        n222 = Bundle(w491, w495) -> (w488:cluster{dbl[], dbl[]})  [unwired: 1 in]
        n223 = Bundle(w491, w490) -> (w489:cluster{dbl[], dbl[]})  [unwired: 1 in]
        n224 = Build Array(w488, w489) -> ()  [unwired: 1 out]
      }
    }
  }
